vi "PathPlanner_PathFinding_SetStartAndGoalPosition.vi"(8 "error in (no error)":errorcluster, 10 "GoalPosition":T1 {"Y" format="%14.3f"; "X" format="%14.3f"}, 11 "StartPosition":T1 {"Y" format="%14.3f"; "X" format="%14.3f"}) -> (0 "error out":errorcluster)   [LabVIEW 2019, in "PathPlanner24.lvlib"]
uses:
  PathPlanner24.lvlib
  <vilib>/Rock Robotics/WPI/ThirdParty/JAS_Junk/TrajLib/TypeDef/TRANSLATION2D.ctl
  ENum/PathPlanner_PathFinding_Cmd_ENUM.ctl
  <vilib>/Rock Robotics/WPI/ThirdParty/JAS_Junk/TrajLib/Translation2d_GetXY.vi
  PathPlanner_GridPosition_New.vi
  PathPlanner_GridPosition_HashCode.vi
  PathPlanner_PathFinder_GetAllNeighbors.vi
  PathPlanner_GridPosition_Get.vi
  PathPlanner_PathFinder_Globals.vi
  <vilib>/Rock Robotics/WPI/ThirdParty/JAS_Junk/TrajLib/Trajectory_Library.lvlib
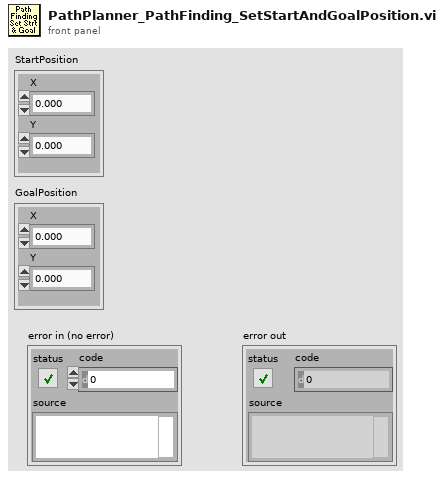
[diagram p1: front panel]
types:
  T1 = typedef "Trajectory_Library.lvlib/TRANSLATION2D.ctl" = cluster{"X":dbl, "Y":dbl}
  T2 = typedef "PathPlanner24.lvlib/PathPlannerFinderGridPosition.ctl" = cluster{"X":i32, "Y":i32}
  T3 = typedef "PathPlanner24.lvlib/PathPlanner_PathFinding_Cmd_ENUM.ctl" = enum16{"Do Nothing", "Reset", "Minor", "Reset and Minor", "Major", "Reset and Major", "Minor and Major", "Reset, Minor, Major"}
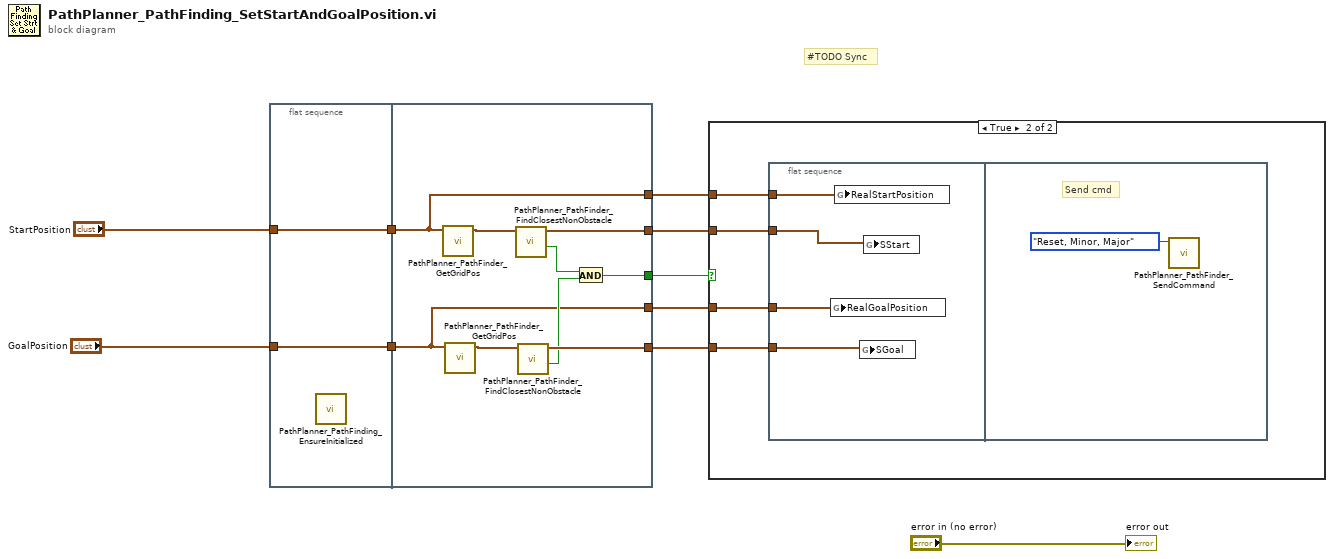
[diagram p0: block diagram]
diagram:
  # "#TODO Sync"
  n1 = flat-sequence {
    tunnel: "GoalPosition" -> [w11]
    tunnel: "StartPosition" -> [w12]
    tunnel: [w12] -> w2
    tunnel: [w11] -> w1
    tunnel: [w20] -> w10
    tunnel: [w18] -> w7
    tunnel: [w17] -> w6
    tunnel: [w14] -> w4
    tunnel: [w13] -> w3
    tunnel: w2 -> [w14]
    tunnel: w1 -> [w13]
    frame #0 {
      n2 = call "PathPlanner_PathFinding_EnsureInitialized.vi"() -> ()  [unwired: 11 in, 1 out]
    }
    frame #1 {
      n3 = call "PathPlanner_PathFinder_GetGridPos.vi"("RealGridPos"=w14) -> ("GridPosition"=w21:T2)  [unwired: 9 in, 1 out]
      n4 = call "PathPlanner_PathFinder_GetGridPos.vi"("RealGridPos"=w13) -> ("GridPosition"=w19:T2)  [unwired: 9 in, 1 out]
      n5 = call "PathPlanner_PathFinder_FindClosestNonObstacle.vi"("GridPosition"=w21) -> ("Found"=w16:bool, "NonObstacleGridPositin"=w20:T2)  [unwired: 9 in]
      n6 = call "PathPlanner_PathFinder_FindClosestNonObstacle.vi"("GridPosition"=w19) -> ("Found"=w15:bool, "NonObstacleGridPositin"=w18:T2)  [unwired: 9 in]
      n7 = And(x=w16, y=w15) -> (x .and. y?=w17:bool)
    }
  }
  n8 = case shown="True" w6 {
    tunnel: w10 -> [_ w25]
    tunnel: w4 -> [_ w24]
    tunnel: w3 -> [_ w23]
    tunnel: w7 -> [_ w22]
    frame False {
      # "Not found\nleave alone"
    }
    frame True {
      n9 = flat-sequence {
        tunnel: w25 -> [w29]
        tunnel: w24 -> [w28]
        tunnel: w23 -> [w27]
        tunnel: w22 -> [w26]
        frame #0 {
          n10 = global write "PathPlanner_PathFinder_Globals.vi" "RealGoalPosition"(w27) -> ()
          n11 = global write "PathPlanner_PathFinder_Globals.vi" "RealStartPosition"(w28) -> ()
          n12 = global write "PathPlanner_PathFinder_Globals.vi" "SGoal"(w26) -> ()
          n13 = global write "PathPlanner_PathFinder_Globals.vi" "SStart"(w29) -> ()
        }
        frame #1 {
          # "Send cmd"
          n14 = call "PathPlanner_PathFinder_SendCommand.vi"("PathFindingCommand"=PathPlanner_PathFinding_Cmd_ENUM."Reset, Minor, Major") -> ()  [unwired: 10 in, 1 out]
        }
      }
    }
  }
  "error out" <- "error in (no error)"
